vi "Get Packed Library Name.vi"(8 "error in (no error)":errorcluster, 11 "PPL in":refnum<class "NI_AB_API_PPL.lvclass">) -> (0 "error out":errorcluster, 2 "Packed library name":string, 3 "PPL out":refnum<class "NI_AB_API_PPL.lvclass">)   [LabVIEW 2020, in "NI_AB_API_PPL.lvclass"]
uses:
  <vilib>/AppBuilder/AB_API/PPL/NI_AB_API_PPL.lvclass
  e:/builds/penguin/labview/branches/2020/dev/dist/vi.lib/AppBuilder/AB_API/Build/NI_AB_API_Build.lvclass
  <vilib>/AppBuilder/AB_Classes/TargetFile/AB_Targetfile.lvclass
  <vilib>/AppBuilder/AB_API/Build/NI_AB_API_Build.lvclass
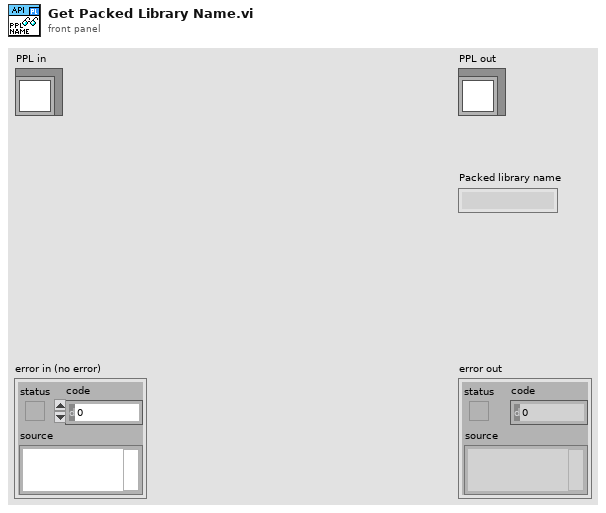
[diagram p1: front panel]
types:
  T1 = typedef "AB_Targetfile.ctl" = cluster{"targetfileName":string, "targetfileGUID":string, "enableDebugging":bool, "versionInfo":cluster{"productName":string, "legalCopyright":string, "companyName":string, "internalName":string, "fileDescription":string}, "eng_consolidatedTypeInfo":string, "fastFileFormat":bool, "eng_LEIFBuildData":u32, "versionIndependent":bool}
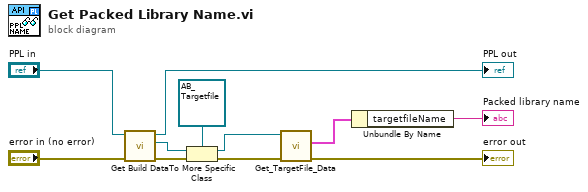
[diagram p0: block diagram]
diagram:
  n1 = call <vilib>:"Get Build Data.vi"("error in (no error)"="error in (no error)", "NI_AB_API_Build in"="PPL in") -> ("error out"=w9:errorcluster, "AB_Build.lvclass"=w6:refnum<class "AB_Build.lvclass">, "NI_AB_API_Build out"=→"PPL out":refnum<class "NI_AB_API_PPL.lvclass">)  [unwired: 7 in]
  n2 = To More Specific Class(target class=refnum<class "AB_Targetfile.lvclass"> refnum ("AB_PackedLibrary in"), reference=w6, error in=w9) -> (specific class reference=w1:refnum<class "AB_Targetfile.lvclass">, error out=w2:errorcluster)
  n3 = call <vilib>:"Get_TargetFile_Data.vi"("error in (no error)"=w2, "AB_Targetfile in"=w1) -> ("error out"=→"error out":errorcluster, "data"=w5:T1)  [unwired: 7 in, 1 out]
  n4 = Unbundle By Name(w5) -> ("targetfileName"=→"Packed library name":string)
